vi "MRayReadShooterCSV.vi"(10 "ShooterFile":string) -> (2 "ShooterArray":dbl[][](array[numeric]))   [LabVIEW 2011]
uses:
  <vilib>/Utility/file.llb/Read From Spreadsheet File (DBL).vi
panel:
  out "Path and file":string
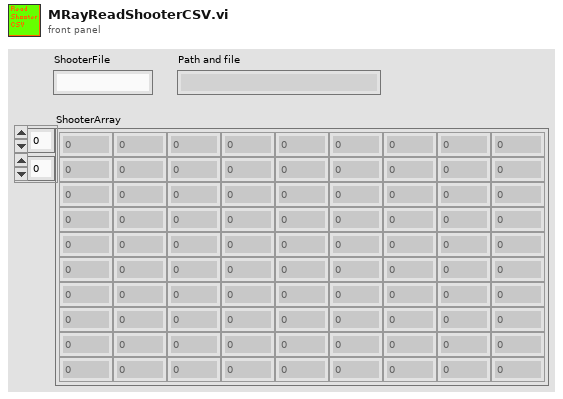
[diagram p1: front panel]
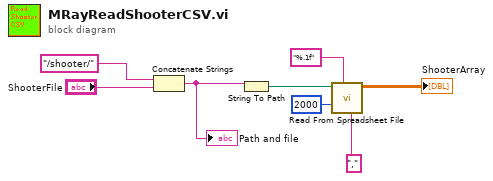
[diagram p0: block diagram]
diagram:
  n1 = Concatenate Strings("/shooter/" ("string"), "ShooterFile") -> (w3:string)
  "Path and file" <- w3
  n2 = String To Path(string=w3) -> (path=w2:path)
  n3 = call-poly <vilib>:"Read From Spreadsheet File.vi"("delimiter (\\t)"="," ("delimiter (\\t)"), "format (%.3f)"="%.1f", "number of rows (all:-1)"=2000, "file path (dialog if empty)"=w2) -> ("all rows"=→"ShooterArray":dbl[][])  [unwired: 1 in, 6 out]
